vi "Fct_Affichage_Data.vi"(4 "Encodeur":string, 5 "Température":string, 6 "Luminosité":string, 7 "Pluiviométrie":string, 9 "Humidité":string, 10 "Direction du vent":string, 11 "Vitesse vent":string) -> (3 "Sortie":string)   [LabVIEW 2017]
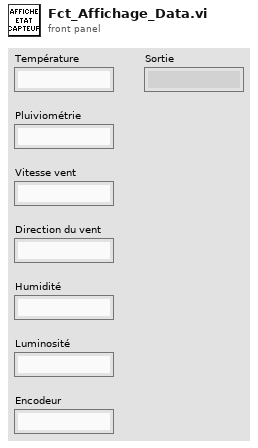
[diagram p1: front panel]
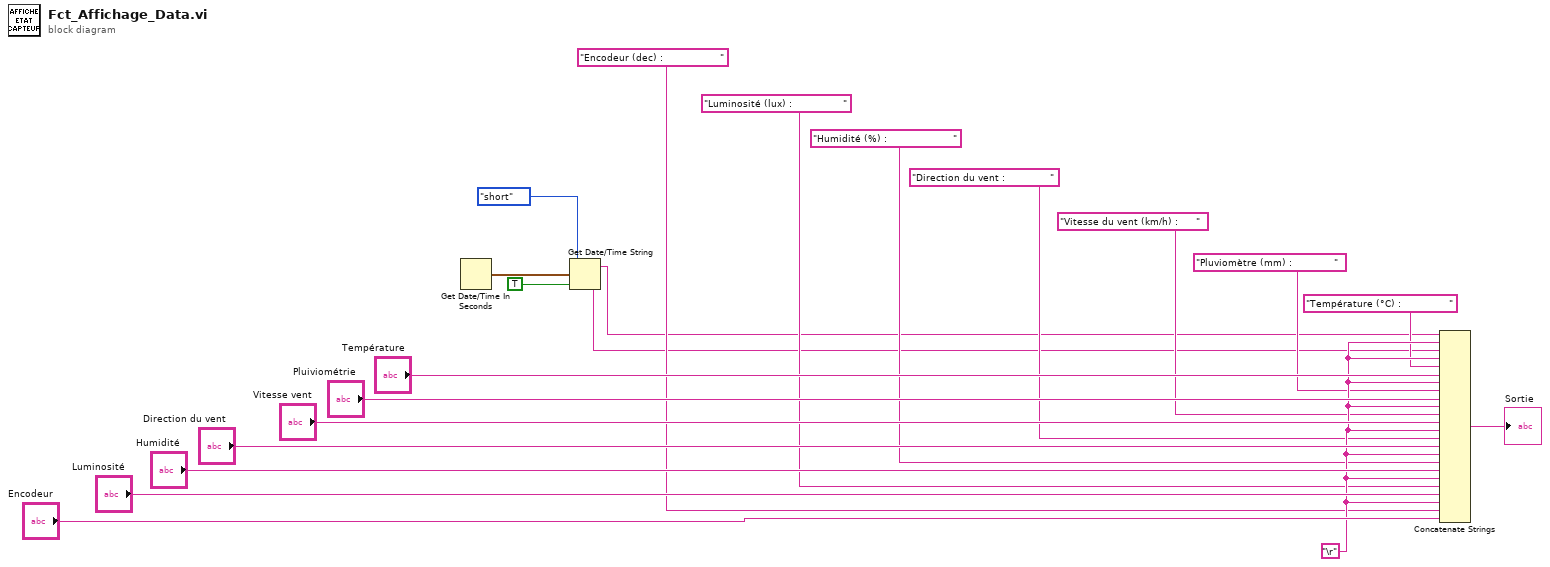
[diagram p0: block diagram]
diagram:
  w14 = "\r"
  n1 = Get Date/Time In Seconds() -> (seconds since 1Jan1904=w2:timestamp)
  n2 = Get Date/Time String(date format (0)=enum16{"short", "long", "abbreviated"}."short" ("format de date (0)"), seconds (now)=w2, want seconds? (F)=TRUE ("secondes ? (F)")) -> (date string=w5:string, time string=w6:string)
  n3 = Concatenate Strings(w5, w14, w6, w14, "Température (°C) :                ", "Température", w14, "Pluviomètre (mm) :              ", "Pluiviométrie", w14, "Vitesse du vent (km/h) :      ", "Vitesse vent", w14, "Direction du vent :               ", "Direction du vent", w14, "Humidité (%) :                      ", "Humidité", w14, "Luminosité (lux) :                 ", "Luminosité", w14, "Encodeur (dec) :                   ", "Encodeur") -> (→"Sortie":string)
